vi "Start Expected Heartbeat Checker.vi"(8 "error in":errorcluster, 10 "Interval":i32, 11 "CANopen Master in":refnum<class "CANopen Master.lvclass">) -> (0 "error out":errorcluster, 3 "CANopen Master out":refnum<class "CANopen Master.lvclass">)   [LabVIEW 2024, in "CANopen Master.lvlib" / "CANopen Master.lvclass"]
uses:
  CANopen Master.lvclass
  CANopen Master.lvclass/CANopen Master.ctl
  Example/Network Management/Network Mangement.lvclass
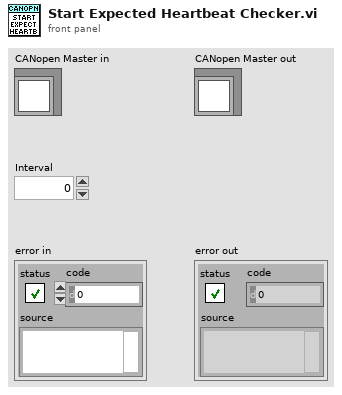
[diagram p1: front panel]
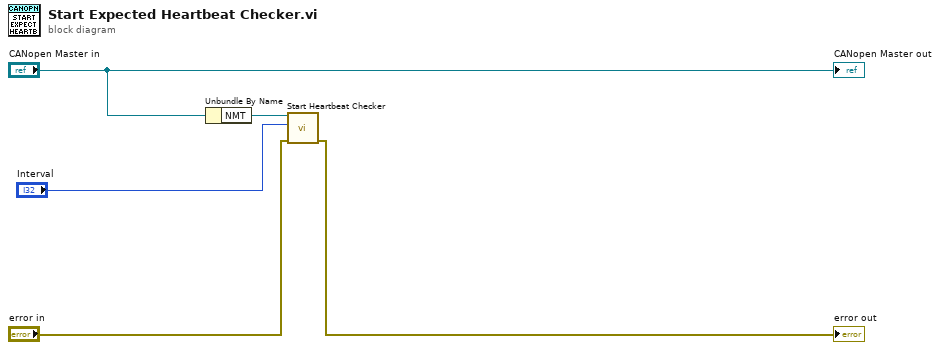
[diagram p0: block diagram]
diagram:
  n1 = Unbundle By Name("CANopen Master in") -> ("NMT"=w4:refnum<class "Network Mangement.lvclass">)
  n2 = call "Start Heartbeat Checker.vi"("Error In"="error in", "Interval"="Interval", "reference in"=w4) -> ("Error Out"=→"error out":errorcluster)  [unwired: 7 in, 1 out]
  "CANopen Master out" <- "CANopen Master in"
